vi "Save BaseNodeType to System Storage File.vi"(8 "error in (no error)":errorcluster, 10 "path":path, 11 "BaseNodeType in":refnum<k39>) -> (0 "error out":errorcluster, 3 "BaseNodeType out":refnum<k39>)   [LabVIEW 2027, in "Custom Device Serialization.lvlib"]
uses:
  Custom Device Serialization.lvlib
  C:/NetCoreDLL/NationalInstruments.VeriStand.SystemStorage.dll
  NetCoreDLL/NationalInstruments.VeriStand.SystemStorage.dll
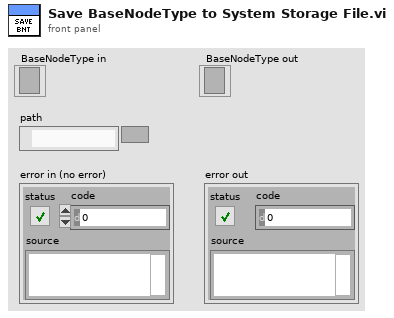
[diagram p1: front panel]
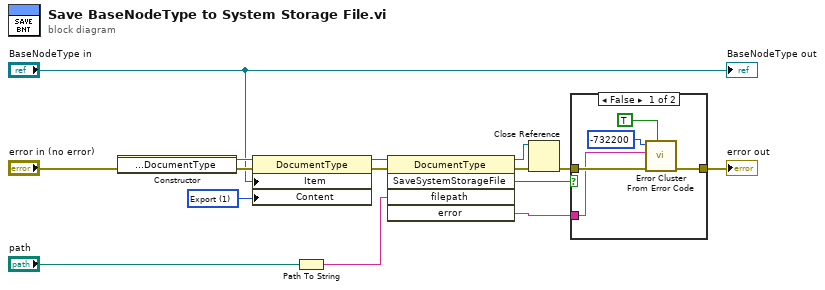
[diagram p0: block diagram]
diagram:
  w14 = 1 items=["Definition", "Export", "SLSC"] ("Content")
  n1 = constructor class="DocumentType"(error in="error in (no error)") -> (reference out=w4:refnum<k39>, error out=w7:errorcluster)  [unwired: 2 in, 1 out]
  n2 = property class="DocumentType"(reference=w4, error in=w7, "Item"="BaseNodeType in", "Content"=w14) -> (reference out=w3:refnum<k39>, error out=w13:errorcluster)
  n3 = Path To String(path="path") -> (string=w2:string)
  n4 = invoke class="DocumentType" method="SaveSystemStorageFile"(reference=w3, error in=w13, "filepath"=w2) -> (reference out=w8:refnum<k39>, error out=w15:errorcluster, "SaveSystemStorageFile"=w9:bool, "error"=w10:string)  [unwired: 2 in, 1 out]
  n5 = Close Reference(reference=w8, error in (no error)=w15) -> (error out=w11:errorcluster)
  n6 = case shown="False" w9 {
    tunnel: [w18 w21] -> w12
    tunnel: w11 -> [w19 w21]
    tunnel: w10 -> [w16 _]
    frame False {
      n7 = call <vilib>:"Error Cluster From Error Code.vi"("show call chain? (False)"=TRUE, "error in (no error)"=w19, "error message (\"\")"=w16, "error code (0)"=-732200) -> ("error out"=w18:errorcluster)  [unwired: 5 in]
    }
    frame True {
    }
  }
  "error out" <- w12
  "BaseNodeType out" <- "BaseNodeType in"
